vi "stopeAO_tt.vi"   [LabVIEW 2013]
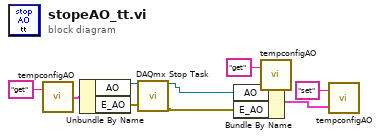
[diagram p0: block diagram]
diagram:
  n1 = call "tempconfigAO.vi"("command"="get") -> ("Temp Config out"=w9:cluster{"AO":refnum<k21>, "E_AO":errorcluster})  [unwired: 1 in]
  n2 = Unbundle By Name(w9) -> ("AO"=w8:refnum<k21>, "E_AO"=w7:errorcluster)
  n3 = call <vilib>:"DAQmx Stop Task.vi"("task/channels in"=w8, "error in"=w7) -> ("task out"=w1:refnum<k21>, "error out"=w2:errorcluster)  [unwired: 12 in]
  n4 = call "tempconfigAO.vi"("command"="get") -> ("Temp Config out"=w4:cluster{"AO":refnum<k21>, "E_AO":errorcluster})  [unwired: 1 in]
  n5 = Bundle By Name(cluster=w4, "AO"=w1, "E_AO"=w2) -> (w3:cluster{"AO":refnum<k21>, "E_AO":errorcluster})
  n6 = call "tempconfigAO.vi"("Temp Config in"=w3, "command"="set") -> ()  [unwired: 1 out]
